vi "SimpleAllign.vi"(0 "y 2":dbl=20.0 format="%#_13g", 1 "y":dbl=0.4 format="%#_13g", 2 "angle":dbl, 4 "Limits tangent":cluster{"output high":dbl, "output low":dbl}={"output high"=1.2, "output low"=-1.2}, 5 "Limits ang":cluster{"output high":dbl, "output low":dbl}={"output high"=1.0, "output low"=-1.0}, 6 "PID gains tangent":T1={"proportional gain (Kc)"=0.0044, "integral time (Ti, min)"=0.0, "derivative time (Td, min)"=-0.085}, 7 "PID gains ang":T1={"proportional gain (Kc)"=0.5, "integral time (Ti, min)"=0.0, "derivative time (Td, min)"=-0.08}, 8 "fc angular":dbl=80.0, 9 "fc tangent":dbl=0.85, 10 "SetPoint":dbl[](array[numeric])=[100.0, 100.0, 0.0], 11 "Position":dbl[](array[numeric])=[208.6539306640625, -200.4281768798828, 3.141592653589793]) -> (3 "Output Vel":dbl[](array[numeric])=[0.0, 0.0, 0.8321627905647668])   [LabVIEW 2018]
uses:
  <vilib>/Analysis/coordinate.llb/Wrap Angle (scalar).vi
  <vilib>/Analysis/_algsub.llb/Real Vector Norm.vi
  <vilib>/Analysis/NI_AAL_Angle.lvlib
  <vilib>/Analysis/NI_AALPro.lvlib
panel:
  out "Angular":dbl(graph)=0.8321627905647668
  out "Tangent":dbl(graph)
  out "NaN":bool
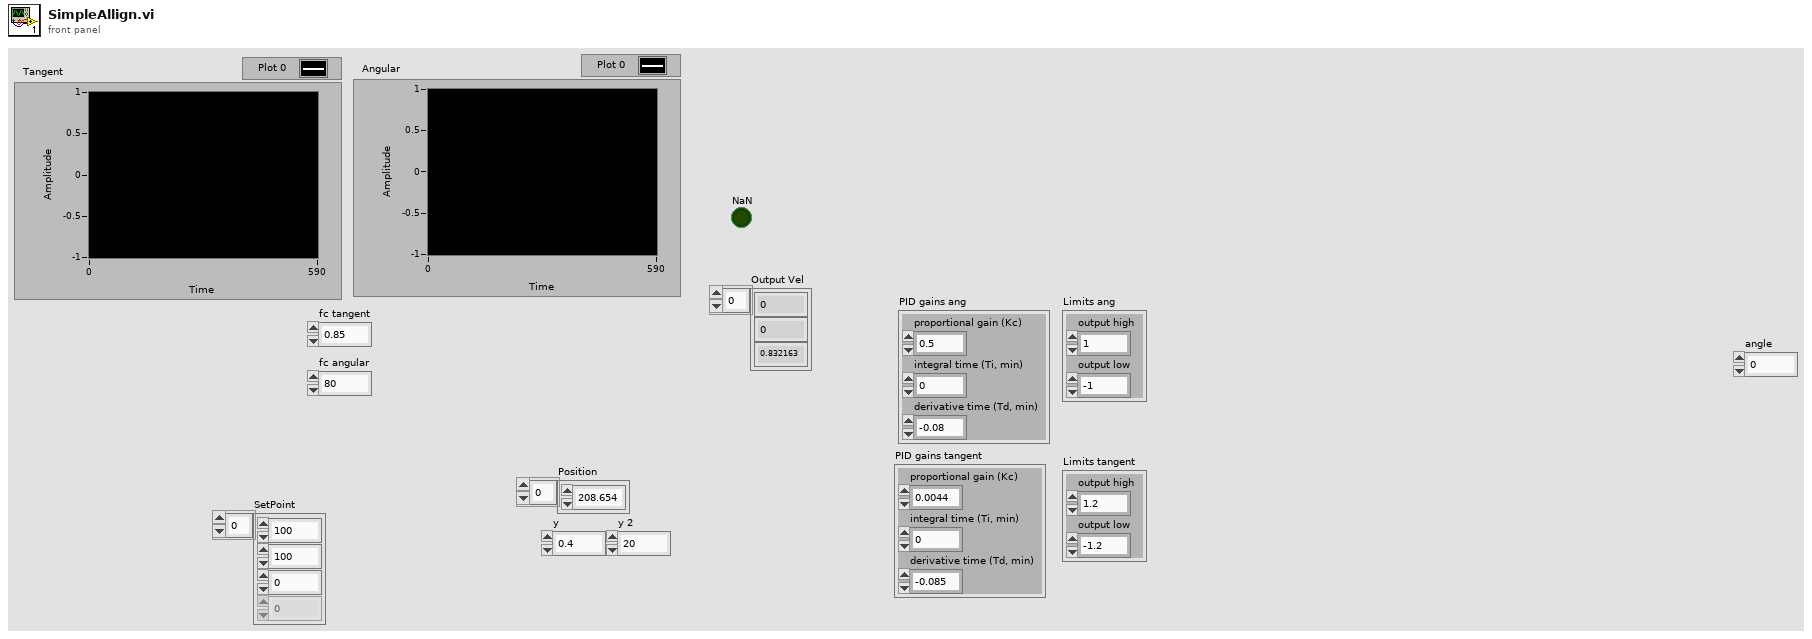
[diagram p1: front panel]
types:
  T1 = cluster{"proportional gain (Kc)":dbl, "integral time (Ti, min)":dbl, "derivative time (Td, min)":dbl}
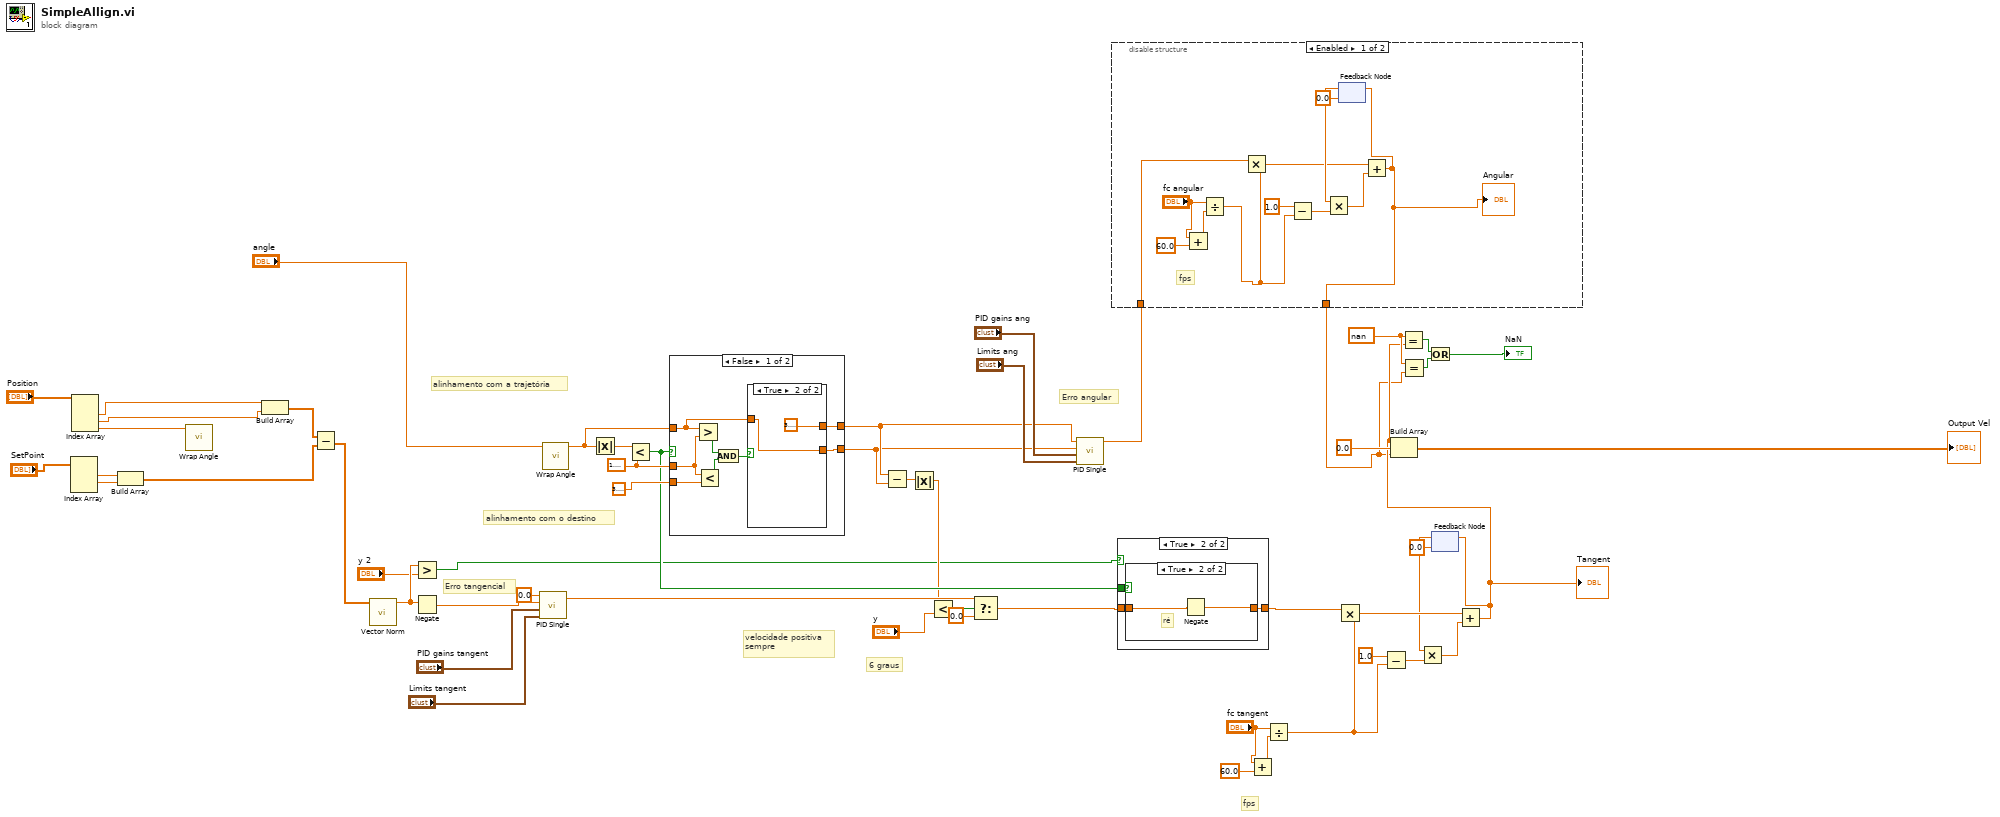
[diagram p0: block diagram]
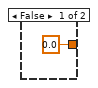
[diagram p3: hidden frame]
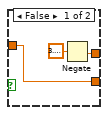
[diagram p5: hidden frame]
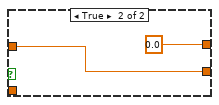
[diagram p6: hidden frame]
diagram:
  w20 = nan
  w35 = 1.5707963267948966
  # "fps"
  # "alinhamento com o destino"
  # "alinhamento com a trajetória"
  # "velocidade positiva\nsempre"
  # "Erro tangencial"
  # "Erro angular"
  # "6 graus"
  n1 = Index Array(array="SetPoint") -> (element #1=w42:dbl, element #2=w41:dbl)  [unwired: 3 in, 1 out]
  n2 = Index Array(array="Position") -> (element #1=w45:dbl, element #2=w44:dbl, element #3=w37:dbl)  [unwired: 3 in]
  n3 = Build Array(w42, w41) -> (w40:dbl[])
  n4 = call-poly <vilib>:"Wrap Angle.vi"("angle in"=w37) -> ()  [unwired: 9 in, 2 out]
  n5 = Build Array(w45, w44) -> (w53:dbl[])
  n6 = Subtract(x=w53, y=w40) -> (x-y=w26:dbl[])
  n7 = call-poly <vilib>:"Vector Norm.vi"("Input Vector"=w26) -> ("norm"=w25:dbl)  [unwired: 9 in, 1 out]
  n8 = Greater?(x=w25, y="y 2") -> (0:w22:bool)
  n9 = Negate(x=w25) -> (-x=w30:dbl)
  n10 = call "PID Single.vi"("Limits"="Limits tangent", "PID gains in"="PID gains tangent", "Variable"=w30, "Setpoint"=0.0) -> ("Out"=w47:dbl)  [unwired: 7 in]
  n11 = call-poly <vilib>:"Wrap Angle.vi"("angle in"="angle") -> ("angle out"=w33:dbl)  [unwired: 9 in, 1 out]
  n12 = Absolute Value(x=w33) -> (abs(x)=w36:dbl)
  n13 = Less?(x=w36, y=w35) -> (x < y?=w31:bool)
  n14 = case shown="False" w31 {
    tunnel: w33 -> [w55 w69]
    tunnel: [w56 w69] -> w28
    tunnel: w35 -> [w62 _]
    tunnel: 3.141592653589793 -> [w61 _]
    tunnel: [w57 0.0 ("Variable")] -> w29
    frame False {
      n15 = Greater?(x=w55, y=w62) -> (0:w59:bool)
      n16 = Less?(x=w62, y=w61) -> (x < y?=w60:bool)
      n17 = And(x=w59, y=w60) -> (x .and. y?=w58:bool)
      n18 = case shown="True" w58 {
        tunnel: [w65 3.141592653589793] -> w57
        tunnel: [w63 w66] -> w56
        tunnel: w55 -> [w63 w66]
        frame False {
          n19 = Negate(x=3.141592653589793) -> (-x=w65:dbl)
        }
        frame True {
        }
      }
    }
    frame True {
    }
  }
  n20 = Subtract(x=w29, y=w28) -> (x-y=w27:dbl)
  n21 = Absolute Value(x=w27) -> (abs(x)=w23:dbl)
  n22 = Less?(x=w23, y="y") -> (x < y?=w48:bool)
  n23 = Select(t=w47, s=w48, f=0.0) -> (s? t:f=w32:dbl)
  n24 = call "PID Single.vi"("Limits"="Limits ang", "PID gains in"="PID gains ang", "Variable"=w28, "Setpoint"=w29) -> ("Out"=w3:dbl)  [unwired: 7 in]
  n25 = disable-structure shown="Enabled" {
    disable-tunnel: [w71 w82] -> w4
    disable-tunnel: w3 -> [w70 w82]
    frame Enabled {
      # "fps"
      n26 = Add(x="fc angular", y=60.0) -> (x+y=w75:dbl)
      n27 = Divide(x="fc angular", y=w75) -> (x/y=w72:dbl)
      n28 = Multiply(x=w70, y=w72) -> (x*y=w76:dbl)
      n29 = Subtract(x=1.0, y=w72) -> (x-y=w78:dbl)
      n30 = feedback #1(0.0) -> (w79:dbl)
      n31 = Multiply(x=w79, y=w78) -> (x*y=w80:dbl)
      n32 = Add(x=w76, y=w80) -> (x+y=w71:dbl)
      "Angular" <- w71
      n33 = feedback-in #1(w71) -> ()
    }
    frame Disabled {
    }
  }
  n34 = case shown="True" w22 {
    tunnel: w32 -> [_ w86]
    tunnel: w31 -> [_ w85]
    tunnel: [0.0 ("f") w84] -> w16
    frame False {
    }
    frame True {
      n35 = case shown="True" w85 {
        tunnel: w86 -> [w87 w89]
        tunnel: [w87 w88] -> w84
        frame False {
        }
        frame True {
          # "ré"
          n36 = Negate(x=w89) -> (-x=w88:dbl)
        }
      }
    }
  }
  n37 = Add(x="fc tangent", y=60.0) -> (x+y=w6:dbl)
  n38 = Divide(x="fc tangent", y=w6) -> (x/y=w9:dbl)
  n39 = Multiply(x=w16, y=w9) -> (x*y=w15:dbl)
  n40 = Subtract(x=1.0, y=w9) -> (x-y=w13:dbl)
  n41 = Equal?(x=w20, y=w4) -> (x = y?=w19:bool)
  n42 = feedback #2(0.0) -> (w12:dbl)
  n43 = Multiply(x=w12, y=w13) -> (x*y=w11:dbl)
  n44 = Add(x=w15, y=w11) -> (x+y=w5:dbl)
  "Tangent" <- w5
  n45 = Build Array(w5, 0.0 ("element"), w4) -> (→"Output Vel":dbl[])
  n46 = Equal?(x=w20, y=w5) -> (x = y?=w18:bool)
  n47 = Or(x=w18, y=w19) -> (x .or. y?=→"NaN":bool)
  n48 = feedback-in #2(w5) -> ()
